vi "RT_mem_i20_vinner(SubVI).vi"(10 "start":bool, 11 "In":dbl format="%#_13g") -> (1 "in_vec":dbl[](array[numeric]), 3 "in_i20":dbl)   [LabVIEW 2011]
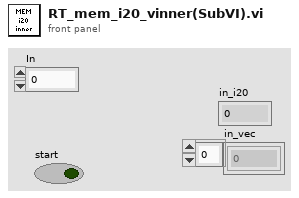
[diagram p1: front panel]
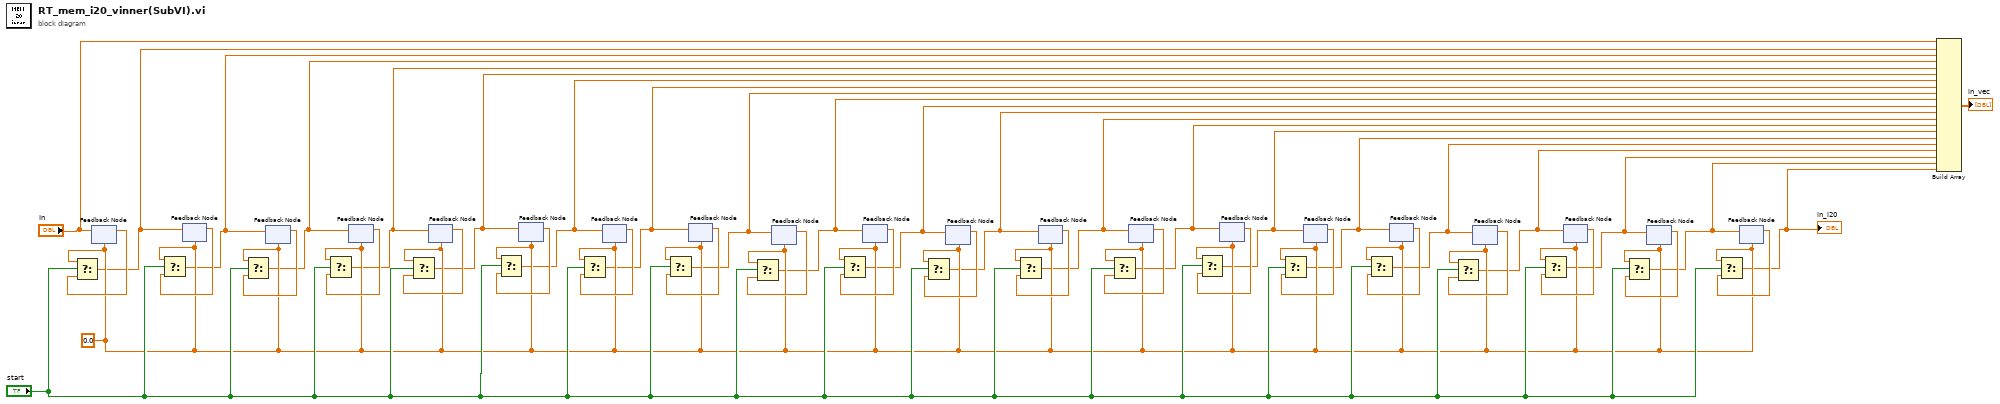
[diagram p0: block diagram]
diagram:
  w23 = 0.0
  n1 = feedback #1(w23) -> (w27:dbl)
  n2 = Select(t=w23, s="start", f=w27) -> (s? t:f=w21:dbl)
  n3 = feedback-in #1("In") -> ()
  n4 = feedback #2(w23) -> (w24:dbl)
  n5 = Select(t=w23, s="start", f=w24) -> (s? t:f=w20:dbl)
  n6 = feedback-in #2(w21) -> ()
  n7 = feedback #3(w23) -> (w25:dbl)
  n8 = Select(t=w23, s="start", f=w25) -> (s? t:f=w19:dbl)
  n9 = feedback-in #3(w20) -> ()
  n10 = feedback #4(w23) -> (w26:dbl)
  n11 = Select(t=w23, s="start", f=w26) -> (s? t:f=w18:dbl)
  n12 = feedback-in #4(w19) -> ()
  n13 = feedback #5(w23) -> (w28:dbl)
  n14 = Select(t=w23, s="start", f=w28) -> (s? t:f=w17:dbl)
  n15 = feedback-in #5(w18) -> ()
  n16 = feedback #6(w23) -> (w31:dbl)
  n17 = Select(t=w23, s="start", f=w31) -> (s? t:f=w16:dbl)
  n18 = feedback-in #6(w17) -> ()
  n19 = feedback #7(w23) -> (w30:dbl)
  n20 = Select(t=w23, s="start", f=w30) -> (s? t:f=w15:dbl)
  n21 = feedback-in #7(w16) -> ()
  n22 = feedback #8(w23) -> (w29:dbl)
  n23 = Select(t=w23, s="start", f=w29) -> (s? t:f=w14:dbl)
  n24 = feedback-in #8(w15) -> ()
  n25 = feedback #9(w23) -> (w35:dbl)
  n26 = Select(t=w23, s="start", f=w35) -> (s? t:f=w13:dbl)
  n27 = feedback-in #9(w14) -> ()
  n28 = feedback #10(w23) -> (w32:dbl)
  n29 = Select(t=w23, s="start", f=w32) -> (s? t:f=w12:dbl)
  n30 = feedback-in #10(w13) -> ()
  n31 = feedback #11(w23) -> (w33:dbl)
  n32 = Select(t=w23, s="start", f=w33) -> (s? t:f=w11:dbl)
  n33 = feedback-in #11(w12) -> ()
  n34 = feedback #12(w23) -> (w34:dbl)
  n35 = Select(t=w23, s="start", f=w34) -> (s? t:f=w10:dbl)
  n36 = feedback-in #12(w11) -> ()
  n37 = feedback #13(w23) -> (w43:dbl)
  n38 = Select(t=w23, s="start", f=w43) -> (s? t:f=w9:dbl)
  n39 = feedback-in #13(w10) -> ()
  n40 = feedback #14(w23) -> (w40:dbl)
  n41 = Select(t=w23, s="start", f=w40) -> (s? t:f=w8:dbl)
  n42 = feedback-in #14(w9) -> ()
  n43 = feedback #15(w23) -> (w41:dbl)
  n44 = Select(t=w23, s="start", f=w41) -> (s? t:f=w7:dbl)
  n45 = feedback-in #15(w8) -> ()
  n46 = feedback #16(w23) -> (w42:dbl)
  n47 = Select(t=w23, s="start", f=w42) -> (s? t:f=w6:dbl)
  n48 = feedback-in #16(w7) -> ()
  n49 = feedback #17(w23) -> (w36:dbl)
  n50 = Select(t=w23, s="start", f=w36) -> (s? t:f=w5:dbl)
  n51 = feedback-in #17(w6) -> ()
  n52 = feedback #18(w23) -> (w39:dbl)
  n53 = Select(t=w23, s="start", f=w39) -> (s? t:f=w4:dbl)
  n54 = feedback-in #18(w5) -> ()
  n55 = feedback #19(w23) -> (w38:dbl)
  n56 = Select(t=w23, s="start", f=w38) -> (s? t:f=w3:dbl)
  n57 = feedback-in #19(w4) -> ()
  n58 = feedback #20(w23) -> (w37:dbl)
  n59 = Select(t=w23, s="start", f=w37) -> (s? t:f=w2:dbl)
  "in_i20" <- w2
  n60 = feedback-in #20(w3) -> ()
  n61 = Build Array("In", w21, w20, w19, w18, w17, w16, w15, w14, w13, w12, w11, w10, w9, w8, w7, w6, w5, w4, w3, w2) -> (→"in_vec":dbl[])
